vi "Read Client Run Vi Path.vi"(8 "error in":errorcluster, 11 "Client Manager in":refnum<class "Client Manager.lvclass">) -> (0 "error out":errorcluster, 2 "Client Run Vi Path":path, 3 "Client Manager out":refnum<class "Client Manager.lvclass">)   [LabVIEW 2014, in "Client Manager.lvclass"]
uses:
  Client Manager.lvclass
  Client Manager.lvclass/Client Manager.ctl
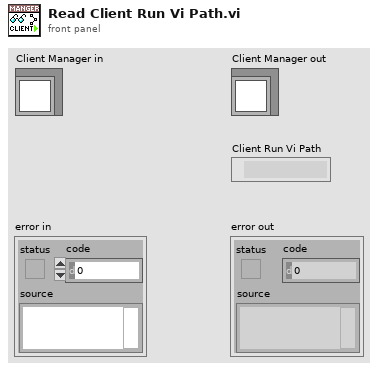
[diagram p1: front panel]
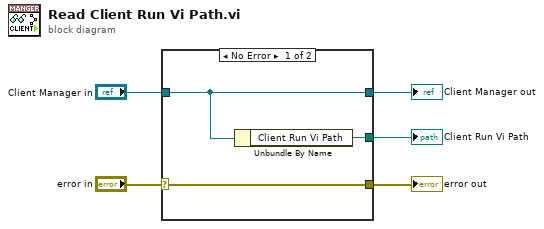
[diagram p0: block diagram]
diagram:
  n1 = case shown="No Error" "error in" {
    selector: "error in" -> [w8 w9]
    tunnel: [w8 w9] -> w4
    tunnel: [w7 w10] -> w2
    tunnel: "Client Manager in" -> [w7 w10]
    tunnel: [w6 _] -> w1
    frame No Error {
      n2 = Unbundle By Name(w7) -> ("Client Run Vi Path"=w6:path)
    }
    frame Error {
    }
  }
  "error out" <- w4
  "Client Manager out" <- w2
  "Client Run Vi Path" <- w1
